vi "picture segmentation.vi"(8 "array lenght (1D)":i32, 9 "y length":i32, 10 "selected image":T1, 11 "x length":i32) -> (3 "chopped image array":picture[][](array[picture]))   [LabVIEW 2014]
uses:
  <vilib>/picture/picture.llb/imagedata.ctl
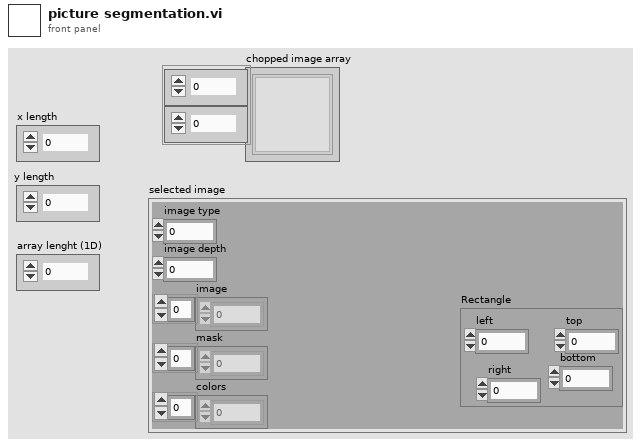
[diagram p1: front panel]
types:
  T1 = typedef "imagedata.ctl" = cluster{"image type":i32, "image depth":i32, "image":u8[], "mask":u8[], "colors":u32[], "Rectangle":cluster{"left":i16, "top":i16, "right":i16, "bottom":i16}}
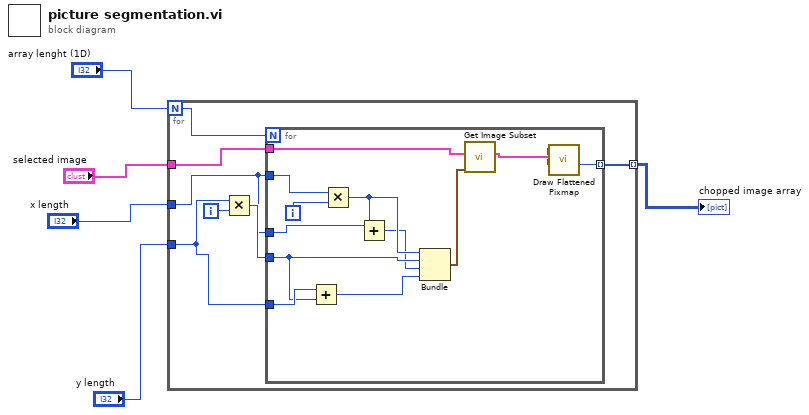
[diagram p0: block diagram]
diagram:
  n1 = for {
    N: "array lenght (1D)" -> [w8]
    tunnel: "x length" -> [w9]
    tunnel: "y length" -> [w10]
    tunnel: "selected image" -> [w12]
    tunnel: [w7] -> w4 mode=indexing
    i -> [w6]
    n2 = Multiply(x=w10, y=w6) -> (x*y=w11:i32)
    n3 = for {
      N: w8 -> [_]
      tunnel: w12 -> [w23]
      tunnel: w11 -> [w19]
      tunnel: w9 -> [w22]
      tunnel: w10 -> [w21]
      tunnel: w9 -> [w20]
      tunnel: [w14] -> w7 mode=indexing
      i -> [w13]
      n4 = Add(x=w21, y=w19) -> (x+y=w16:i32)
      n5 = Multiply(x=w22, y=w13) -> (x*y=w18:i32)
      n6 = Add(x=w20, y=w18) -> (x+y=w17:i32)
      n7 = Bundle(w18, w19, w17, w16) -> (w15:cluster{i32, i32, i32, i32})  [unwired: 1 in]
      n8 = call <vilib>:"Get Image Subset.vi"("subset rect"=w15, "image data"=w23) -> ("image subset"=w24:T1)  [unwired: 4 in, 1 out]
      n9 = call <vilib>:"Draw Flattened Pixmap.vi"("image data"=w24) -> ("new picture"=w14:picture)  [unwired: 8 in]
    }
  }
  "chopped image array" <- w4
